vi "mav_connection_close.vi"(8 "error in":errorcluster, 9 "connection_type":enum16{"SERIAL", "TCP", "UDP"}(ring), 11 "mav_connection_in":T1) -> (0 "error out":errorcluster)   [LabVIEW 2023]
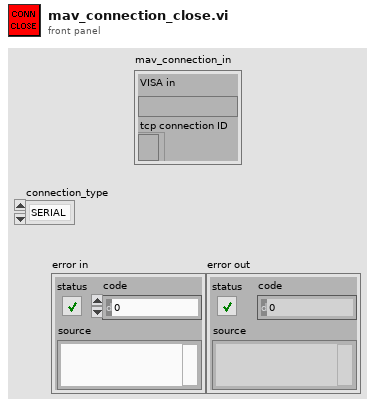
[diagram p1: front panel]
types:
  T1 = cluster{"VISA in":refnum<visa-resource-name>, "tcp connection ID":refnum<k5>}
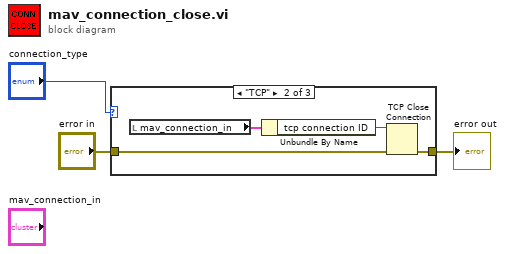
[diagram p0: block diagram]
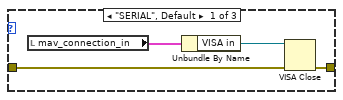
[diagram p2: hidden frame]
diagram:
  n1 = case shown="\"TCP\"" "connection_type" {
    tunnel: "error in" -> [w7 w11 w12]
    tunnel: [w6 w10 w12] -> w2
    frame "SERIAL", Default {
      n2 = local read "mav_connection_in"() -> (w5:T1)
      n3 = Unbundle By Name(w5) -> ("VISA in"=w4:refnum<visa-resource-name>)
      n4 = VISA Close(VISA resource name=w4, error in (no error)=w7) -> (error out=w6:errorcluster)
    }
    frame "TCP" {
      n5 = local read "mav_connection_in"() -> (w9:T1)
      n6 = Unbundle By Name(w9) -> ("tcp connection ID"=w8:refnum<k5>)
      n7 = TCP Close Connection(connection ID=w8, error in (no error)=w11) -> (error out=w10:errorcluster)  [unwired: 1 in, 1 out]
    }
    frame "UDP" {
    }
  }
  "error out" <- w2
